vi "Create Frame Pattern Script.vi"(8 "error in (no error)":errorcluster, 9 "ChipID":u8, 10 "Frame_Data":T1={"Pattern_Name"="", "Operation Mode"=enum."Normal", "BurstLength"=enum."0", "FSN"=0, "Start_Addr"=0, "Data"=[], "R/W?"=enum."Read", "Opcode"=[], "ChipID"=1, "num of wait cycle of read"=0} {"Data" format="%x"; "Start_Addr" format="%x"}, 11 "BML_Frame_ReadData_ValueCap in":refnum<class "BML_Frame_ReadData_ValueCap.lvclass">) -> (0 "error out":errorcluster, 3 "BML_Frame_ReadData_ValueCap out":refnum<class "BML_Frame_ReadData_ValueCap.lvclass">)   [LabVIEW 2018, in "BML_Frame_ReadData_ValueCap.lvclass"]
uses:
  BML_Frame_ReadData_ValueCap.lvclass
  C:/P4 Workspace/PC Client/Solutions/5g_eap/HiSi/trunk/1.0/BML_Pattern_Gen_Refactor/Classes/BML_Frame_Root/BML_Frame_Root.lvclass
  Config_Read/Frame_Data.ctl
  Config_Read/OperationMode.ctl
  Config_Read/BurstLength.ctl
  Config_Read/RW_Option.ctl
  BML_Frame_ReadData_ValueCap.lvclass/BML_Frame_ReadData_ValueCap.ctl
  BML_Frame_Root/BML_Frame_Root.lvclass/BML_Frame_Root.ctl
  BML_Frame_Cmd/BML_Frame_Command.lvclass
  BML_Frame_Addr/BML_Frame_Addr.lvclass
  Config_Read/Config_Read_BML.lvclass
  BML_Frame_Root/BML_Frame_Root.lvclass
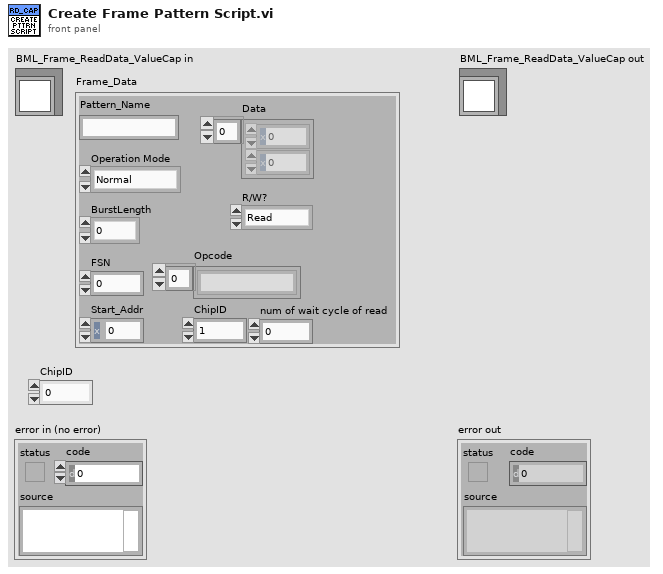
[diagram p1: front panel]
types:
  T1 = typedef "Config_Read_BML.lvclass/Frame_Data.ctl" = cluster{"Pattern_Name":string, "Operation Mode":T2, "BurstLength":T3, "FSN":u8, "Start_Addr":u16, "Data":u8[], "R/W?":T4, "Opcode":string[], "ChipID":u8, "num of wait cycle of read":i8}
  T2 = typedef "Config_Read_BML.lvclass/OperationMode.ctl" = enum8{"Normal", "ImmeEffect", "InitSlaveID", "LoadData"}
  T3 = typedef "Config_Read_BML.lvclass/BurstLength.ctl" = enum8{"0", "2", "3", "4", "5", "8", "16", "32"}
  T4 = typedef "Config_Read_BML.lvclass/RW_Option.ctl" = enum16{"Read", "Write", "R/W"}
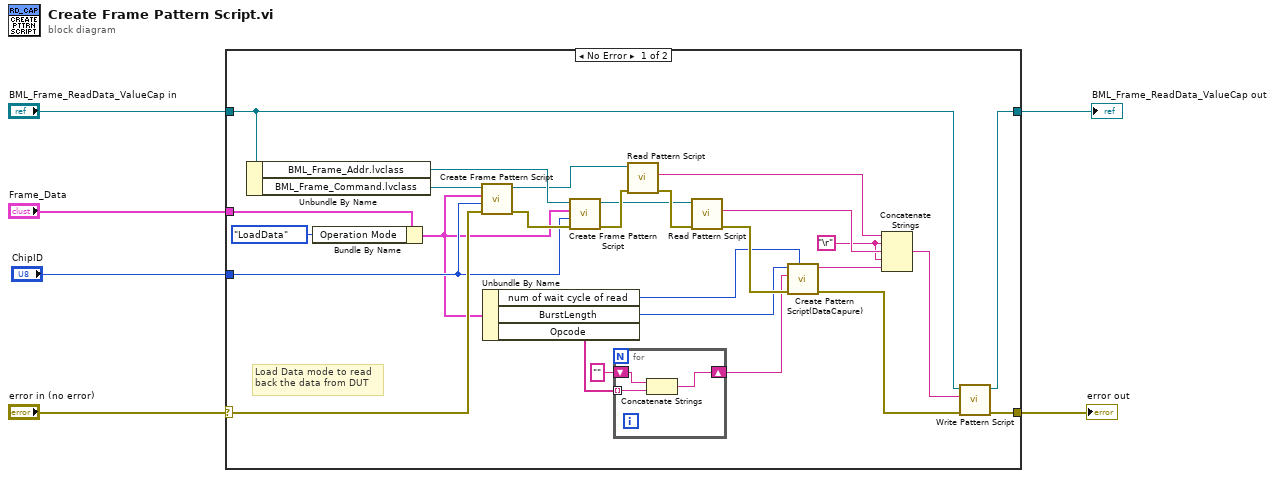
[diagram p0: block diagram]
diagram:
  n1 = case shown="No Error" "error in (no error)" {
    selector: "error in (no error)" -> [w30 w37]
    tunnel: "BML_Frame_ReadData_ValueCap in" -> [w17 w38]
    tunnel: [w16 w38] -> w2
    tunnel: [w18 w37] -> w1
    tunnel: "Frame_Data" -> [w33 _]
    tunnel: "ChipID" -> [w27 _]
    frame No Error {
      w15 = "\r"
      # "Load Data mode to read\nback the data from DUT"
      n2 = Unbundle By Name(w17) -> ("BML_Frame_Addr.lvclass"=w29:refnum<class "BML_Frame_Addr.lvclass">, "BML_Frame_Command.lvclass"=w31:refnum<class "BML_Frame_Command.lvclass">)
      n3 = Bundle By Name(cluster=w33, "Operation Mode"=OperationMode."LoadData") -> (w22:T1)
      n4 = call-dynamic "Create Frame Pattern Script.vi"("error in (no error)"=w30, "ChipID"=w27, "Frame_Data"=w22, "BML_Frame_Command in"=w31) -> ("error out"=w28:errorcluster, "BML_Frame_Command out"=w26:refnum<class "BML_Frame_Command.lvclass">)  [unwired: 6 in]
      n5 = Unbundle By Name(w22) -> ("num of wait cycle of read"=w7:i8, "BurstLength"=w11:T3, "Opcode"=w10:string[])
      n6 = call-dynamic "Create Frame Pattern Script.vi"("error in (no error)"=w28, "ChipID"=w27, "Frame_Data"=w22, "BML_Frame_Addr in"=w29) -> ("error out"=w25:errorcluster, "BML_Frame_Addr out"=w23:refnum<class "BML_Frame_Addr.lvclass">)  [unwired: 6 in]
      n7 = for {
        tunnel: w10 -> [w36] mode=indexing
        shift-right: [w35] -> w8
        shift-left: "" -> [w34]
        n8 = Concatenate Strings(w34, w36) -> (w35:string)
      }
      n9 = call "Read Pattern Script.vi"("error in (no error)"=w25, "BML_Frame_Root in"=w26) -> ("error out"=w24:errorcluster, "Pattern Script"=w21:string)  [unwired: 7 in, 1 out]
      n10 = call "Read Pattern Script.vi"("error in (no error)"=w24, "BML_Frame_Root in"=w23) -> ("error out"=w14:errorcluster, "Pattern Script"=w20:string)  [unwired: 7 in, 1 out]
      n11 = call "Create Pattern Script(DataCapure).vi"("Num of Cycles"=w7, "error in (no error)"=w14, "Opcode"=w8, "BurstLength"=w11) -> ("error out"=w12:errorcluster, "String"=w13:string)  [unwired: 6 in]
      n12 = Concatenate Strings(w21, w15, w20, w15, w13) -> (w19:string)
      n13 = call "Write Pattern Script.vi"("error in (no error)"=w12, "Pattern Script"=w19, "BML_Frame_Root in"=w17) -> ("error out"=w18:errorcluster, "BML_Frame_Root out"=w16:refnum<class "BML_Frame_ReadData_ValueCap.lvclass">)  [unwired: 7 in]
    }
    frame Error {
    }
  }
  "error out" <- w1
  "BML_Frame_ReadData_ValueCap out" <- w2
